vi "Find Package By Name.vi"(10 "Package Name":string, 11 "Packages":refnum<class "Package.lvclass">[](array[class])) -> (1 "Index":i32, 2 "Found?":bool, 3 "Package out":refnum<class "Package.lvclass">)   [LabVIEW 2016, in "Packages.lvlib"]
uses:
  Packages.lvlib
  Package_class/Package.lvclass
  Package_class/Package.lvclass/Package.ctl
  Package_class/Read Name.vi
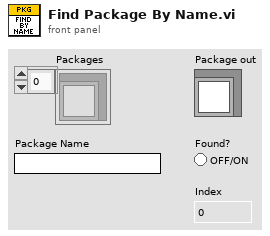
[diagram p1: front panel]
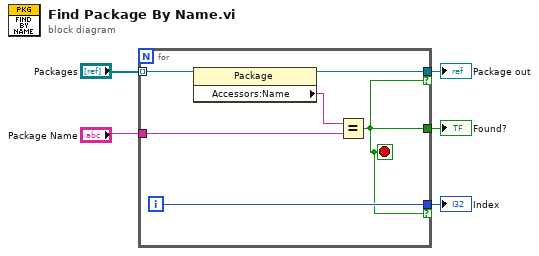
[diagram p0: block diagram]
diagram:
  n1 = for {
    tunnel: "Packages" -> [w11] mode=indexing
    tunnel: [w10] -> w2 if=w6
    tunnel: "Package Name" -> [w8]
    tunnel: [w6] -> w3
    tunnel: [w7] -> w1 if=w6
    i -> [w7]
    stop <- w6 stop-if-true
    n2 = property class="Package"(reference=w11) -> (reference out=w10:refnum<class "Package.lvclass">, "Accessors:Name"=w9:string)  [unwired: 1 in, 1 out]
    n3 = Equal?(x=w9, y=w8) -> (x = y?=w6:bool)
  }
  "Found?" <- w3
  "Package out" <- w2
  "Index" <- w1
